vi "Stop Test Engine Actor.vi"(8 "error in (no error)":errorcluster, 11 "TestBench in":refnum<class "TestBench.lvclass">) -> (0 "error out":errorcluster, 3 "TestBench out":refnum<class "TestBench.lvclass">)   [LabVIEW 2019, in "TestBench.lvlib" / "TestBench.lvclass"]
uses:
  TestBench.lvclass
  C:/Program Files (x86)/National Instruments/LabVIEW 2019/vi.lib/ActorFramework/Actor/Actor.lvclass
  <vilib>/ActorFramework/Actor/Actor.lvclass/Actor.ctl
  <vilib>/ActorFramework/Message Enqueuer/Message Enqueuer.lvclass/Message Enqueuer.ctl
  TestBench.lvclass/TestBench.ctl
  <vilib>/NI/Event Source Actor/Event Source/Event Source Messages/Unregister Msg/Unregister Msg.lvclass/Unregister Msg.ctl
  <vilib>/ActorFramework/Message Enqueuer/Init from Existing Queue.vi
  <vilib>/ActorFramework/Message Enqueuer/Enqueue.vi
  <vilib>/NI/Event Source Actor/Event Source/Event Source Messages/Unregister Msg/Unregister Msg.lvclass
  C:/Program Files (x86)/National Instruments/LabVIEW 2019/vi.lib/ActorFramework/Message/Message.lvclass
  <vilib>/ActorFramework/Stop Msg/Stop Msg.lvclass
  <vilib>/ActorFramework/Message Priority Queue/Priority Enqueue.vi
  <vilib>/ActorFramework/Message Enqueuer/Message Enqueuer.lvclass
  <vilib>/ActorFramework/Actor/Actor.lvclass
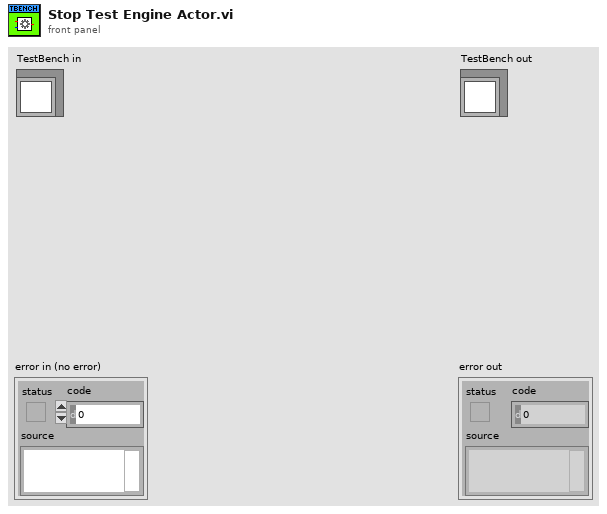
[diagram p1: front panel]
types:
  T1 = map{string, refnum<class "Message Enqueuer.lvclass">}
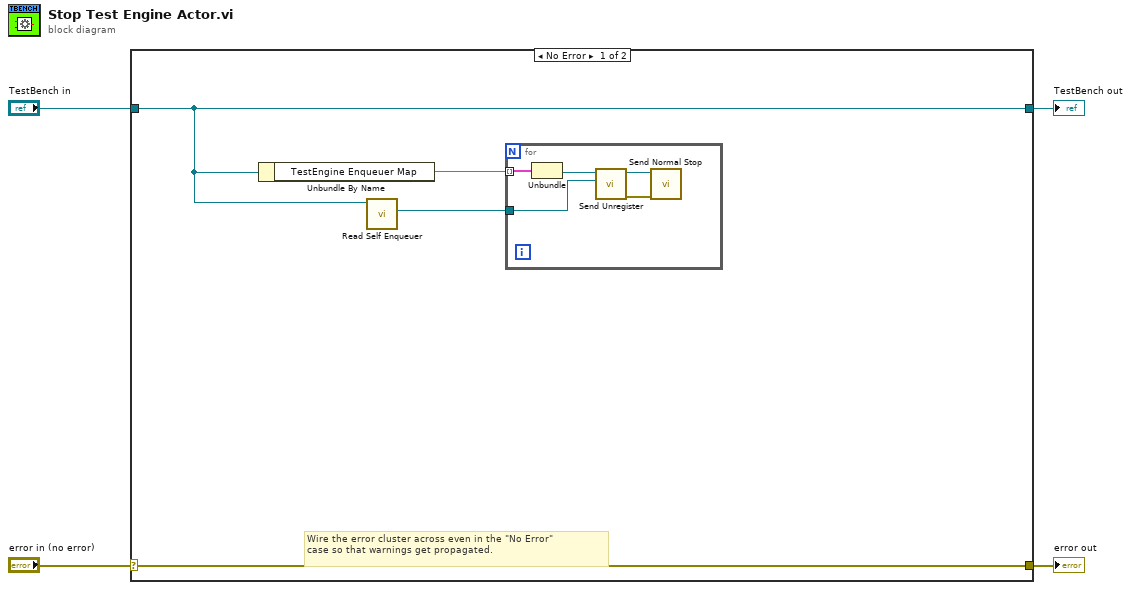
[diagram p0: block diagram]
diagram:
  n1 = case shown="No Error" "error in (no error)" {
    selector: "error in (no error)" -> [w8 w15]
    tunnel: [w8 w15] -> w3
    tunnel: [w6 w14] -> w1
    tunnel: "TestBench in" -> [w6 w14]
    frame No Error {
      # "Wire the error cluster across even in the \"No Error\"\ncase so that warnings get propagated."
      n2 = Unbundle By Name(w6) -> ("TestEngine Enqueuer Map"=w7:T1)
      n3 = call <vilib>:"Read Self Enqueuer.vi"("Actor"=w6) -> ("Self Enqueuer"=w5:refnum<class "Message Enqueuer.lvclass">)  [unwired: 10 in]
      n4 = for {
        tunnel: w7 -> [w13] mode=indexing
        tunnel: w5 -> [w9]
        n5 = Unbundle(w13) -> ("TestEngine Actor's Enqueuer"=w12:refnum<class "Message Enqueuer.lvclass">)  [unwired: 1 out]
        n6 = call <vilib>:"Send Unregister.vi"("Registrant Address"=w9, "Event Source Address"=w12) -> ("Error Out"=w10:errorcluster, "Event Source Address Out"=w11:refnum<class "Message Enqueuer.lvclass">)  [unwired: 8 in]
        n7 = call <vilib>:"Send Normal Stop.vi"("error in (no error)"=w10, "Message Enqueuer"=w11) -> ()  [unwired: 9 in, 1 out]
      }
    }
    frame Error {
    }
  }
  "error out" <- w3
  "TestBench out" <- w1
